vi "Set Metadata Properties.vi"(8 "error in (no error)":errorcluster, 10 "Properties":T1[](array[typedef]), 11 "CycloneDX SBOM in":refnum<class "CycloneDX SBOM.lvclass">) -> (0 "error out":errorcluster, 3 "CycloneDX SBOM out":refnum<class "CycloneDX SBOM.lvclass">)   [LabVIEW 2017, in "LabVIEW CycloneDX SBOM.lvlib" / "CycloneDX SBOM.lvclass"]
doc: "Set metadata properties of the SBOM."
uses:
  CycloneDX SBOM.lvclass
  C:/LabVIEW Working Directory/labview-cyclonedx-sbom/Source/CycloneDX/CycloneDX JSON/CycloneDX JSON.lvclass
  CycloneDX JSON/Name Value Pair.ctl
  CycloneDX JSON/CycloneDX JSON.lvclass
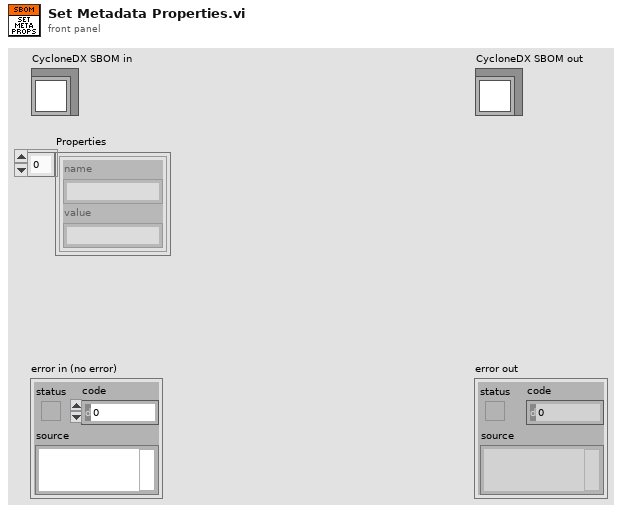
[diagram p1: front panel]
types:
  T1 = typedef "LabVIEW CycloneDX SBOM.lvlib/CycloneDX JSON.lvclass/Name Value Pair.ctl" = cluster{"name":string, "value":string}
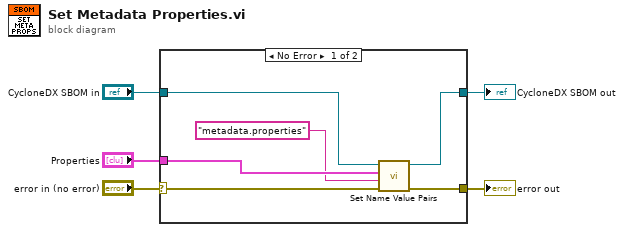
[diagram p0: block diagram]
diagram:
  n1 = case shown="No Error" "error in (no error)" {
    selector: "error in (no error)" -> [w10 w12]
    tunnel: [w11 w12] -> w5
    tunnel: [w9 w13] -> w3
    tunnel: "CycloneDX SBOM in" -> [w8 w13]
    tunnel: "Properties" -> [w7 _]
    frame No Error {
      n2 = call "Set Name Value Pairs.vi"("error in (no error)"=w10, "Object (or Item) Path"="metadata.properties", "Properties"=w7, "CycloneDX JSON in"=w8) -> ("error out"=w11:errorcluster, "CycloneDX JSON out"=w9:refnum<class "CycloneDX SBOM.lvclass">)  [unwired: 6 in]
    }
    frame Error {
    }
  }
  "error out" <- w5
  "CycloneDX SBOM out" <- w3
